vi "energisation rate.vi"(8 "waittime":dbl, 9 "actual field":dbl, 10 "B-Field (goto)":dbl) -> (1 "wait":dbl, 2 "new field":dbl)   [LabVIEW 2010]
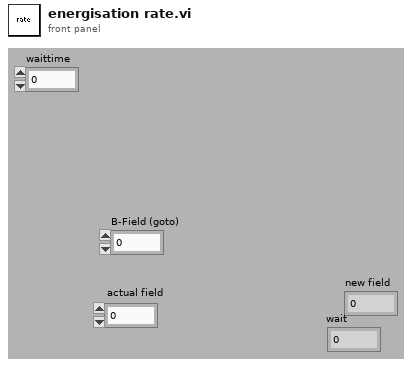
[diagram p1: front panel]
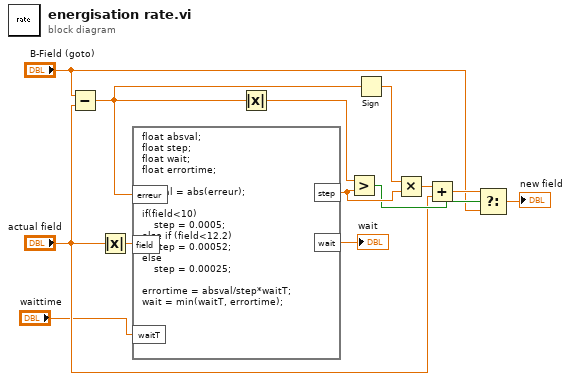
[diagram p0: block diagram]
diagram:
  n1 = Subtract(x="B-Field (goto)", y="actual field") -> (x-y=w3:dbl)
  n2 = Absolute Value(x="actual field") -> (abs(x)=w11:dbl)
  n3 = formula code="float absval;\nfloat step;\nfloat wait;\nfloat errortime;\n\nabsval = abs(erreur);\n\nif(field<10)\n    step = 0.0005;\nelse if (field<12.2)\n    step = 0.00052;\nelse\n    step = 0.00025;\n\nerrortime = absval/step*waitT;\nwait = min(waitT, errortime);"("field"=w11, "erreur"=w3, "waitT"="waittime") -> ("step"=w6:dbl, "wait"=→"wait":dbl)
  n4 = Absolute Value(x=w3) -> (abs(x)=w8:dbl)
  n5 = Greater?(x=w8, y=w6) -> (0:w5:bool)
  n6 = Sign(1:w3) -> (0:w9:dbl)
  n7 = Multiply(x=w9, y=w6) -> (x*y=w13:dbl)
  n8 = Add(x=w13, y="actual field") -> (x+y=w12:dbl)
  n9 = Select(t=w12, s=w5, f="B-Field (goto)") -> (s? t:f=→"new field":dbl)
